vi "Read plots names.vi"(8 "error in (no error)":errorcluster, 10 "Combo Box":string(combo)="Spectra", 11 "Control-Client in":refnum<class "Control-Client.lvclass">) -> (0 "error out":errorcluster, 2 "Plots names":string[](array[string])=["part", "full"], 3 "Control-Client out":refnum<class "Control-Client.lvclass">)   [LabVIEW 2019, in "Control-Client.lvclass"]
uses:
  Control-Client.lvclass
  Control-Client.lvclass/Control-Client.ctl
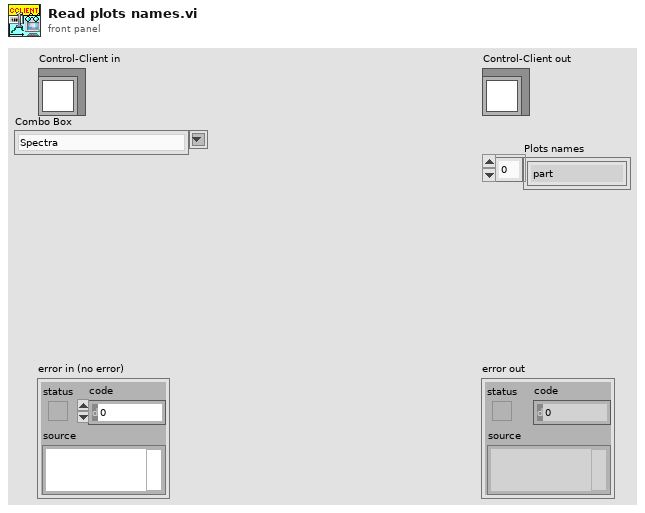
[diagram p1: front panel]
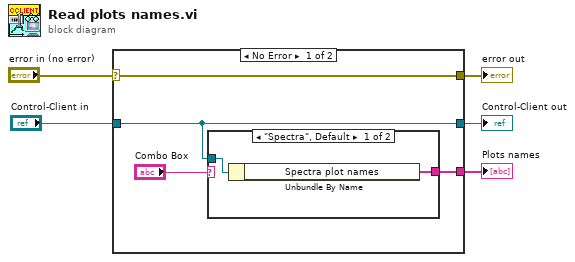
[diagram p0: block diagram]
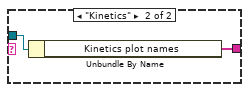
[diagram p2: hidden frame]
diagram:
  n1 = case shown="No Error" "error in (no error)" {
    selector: "error in (no error)" -> [w9 w14]
    tunnel: [w9 w14] -> w4
    tunnel: [w8 w15] -> w2
    tunnel: "Control-Client in" -> [w8 w15]
    tunnel: [w7 _] -> w1
    frame No Error {
      n2 = case shown="\"Spectra\", Default" "Combo Box" {
        tunnel: w8 -> [w11 w13]
        tunnel: [w10 w12] -> w7
        frame "Spectra", Default {
          n3 = Unbundle By Name(w11) -> ("Spectra plot names"=w10:string[])
        }
        frame "Kinetics" {
          n4 = Unbundle By Name(w13) -> ("Kinetics plot names"=w12:string[])
        }
      }
    }
    frame Error {
    }
  }
  "error out" <- w4
  "Control-Client out" <- w2
  "Plots names" <- w1
